vi "Auto Scale.vi"(8 "error in (no error)":errorcluster, 10 "Scale (X AND Y)":enum16{"X AND Y", "X", "Y", "NONE"}(ring), 11 "Graph Manager in":refnum<class "Graph Manager.lvclass">) -> (0 "error out":errorcluster, 3 "Graph Manager out":refnum<class "Graph Manager.lvclass">)   [LabVIEW 2016, in "Graph Manager.lvclass"]
uses:
  Graph Manager.lvclass
  Graph Manager.lvclass/Graph Manager.ctl
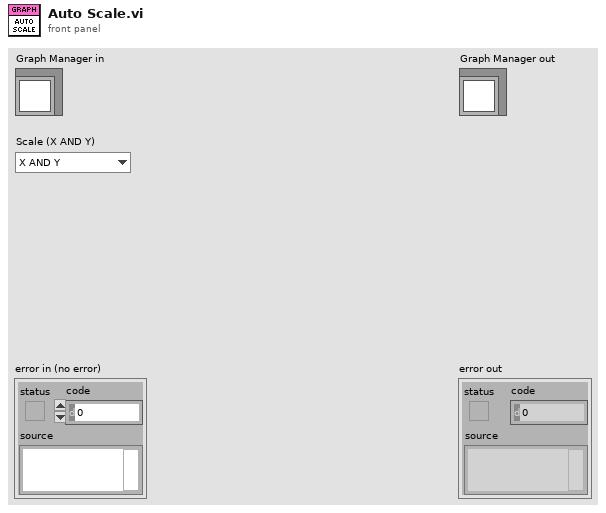
[diagram p1: front panel]
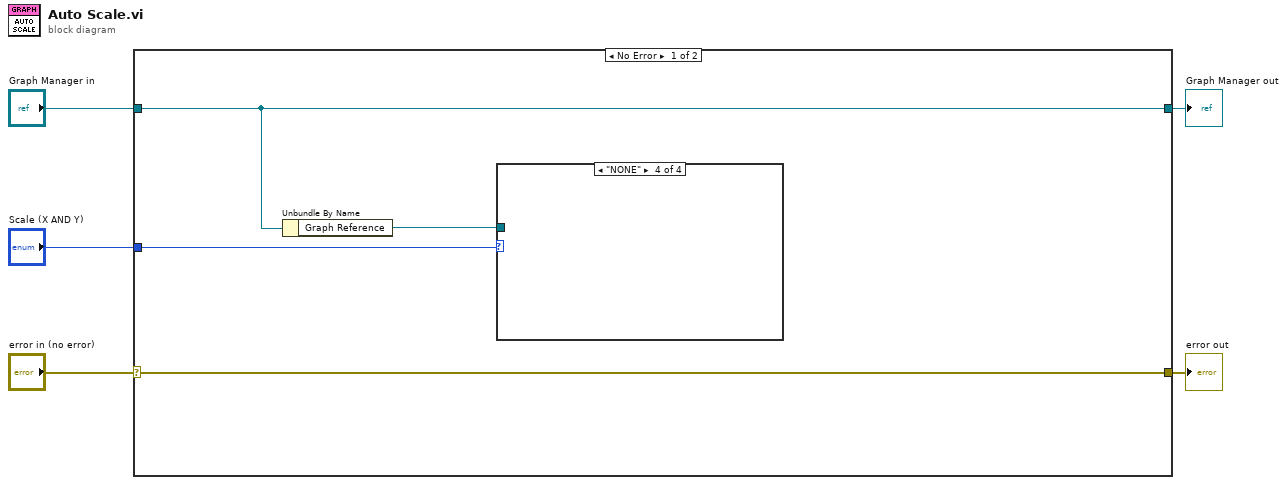
[diagram p0: block diagram]
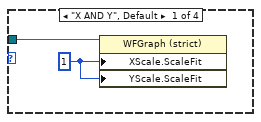
[diagram p2: hidden frame]
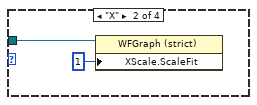
[diagram p3: hidden frame]
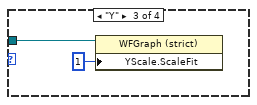
[diagram p4: hidden frame]
diagram:
  n1 = case shown="No Error" "error in (no error)" {
    selector: "error in (no error)" -> [w9 w17]
    tunnel: [w9 w17] -> w4
    tunnel: [w8 w16] -> w2
    tunnel: "Graph Manager in" -> [w8 w16]
    tunnel: "Scale (X AND Y)" -> [w6 _]
    frame No Error {
      n2 = Unbundle By Name(w8) -> ("Graph Reference"=w7:refnum<vi>)
      n3 = case shown="\"NONE\"" w6 {
        tunnel: w7 -> [w11 w12 w14 _]
        frame "X AND Y", Default {
          w10 = u8 1 ("X Scale.Scale Fit")
          n4 = property class="WFGraph (strict)"(reference=w11, "XScale.ScaleFit"=w10, "YScale.ScaleFit"=w10) -> ()  [unwired: 1 in, 2 out]
        }
        frame "X" {
          n5 = property class="WFGraph (strict)"(reference=w12, "XScale.ScaleFit"=u8 1 ("X Scale.Scale Fit")) -> ()  [unwired: 1 in, 2 out]
        }
        frame "Y" {
          n6 = property class="WFGraph (strict)"(reference=w14, "YScale.ScaleFit"=u8 1 ("X Scale.Scale Fit")) -> ()  [unwired: 1 in, 2 out]
        }
        frame "NONE" {
        }
      }
    }
    frame Error {
    }
  }
  "error out" <- w4
  "Graph Manager out" <- w2
